vi "Channel RED.vi"() -> ()   [LabVIEW 2012]
uses:
  RxTXCamera/RxTxCamera.lvclass
  CCDCamera/CCDCamera.lvclass
  RxTx/RxTx.lvclass/RxTx.ctl
  CCDCamera/CCDCamera.lvclass/CCDCamera.ctl
  RxTXCamera/RxTxCamera.lvclass/RxTxCamera.ctl
  RxTx/Read Message.vi
  RxTXCamera/Read Construct String Header.lvclass.vi
  RxTXCamera/Write Construct String Header.lvclass.vi
  RxTXCamera/Read Construct String Setup Cam.lvclass.vi
  RxTXCamera/Write Construct String Setup Cam.lvclass.vi
  Construct String Header/Read Header Contents.vi
  Construct String Setup Cam/Read Camera Setup.vi
  Construct String Header/Construct String Header.lvclass
  Construct String Setup Cam/Construct String Setup Cam.lvclass
  RxTx/RxTx.lvclass
  Cooler/Cooler.lvclass
panel:
  in  "RxTxCamera.lvclass":refnum<class "RxTxCamera.lvclass">
  in  "error out":errorcluster
  in  "Instrument out":refnum<class "CCDCamera.lvclass">
  in  "RxTxCamera.lvclass 2":refnum<class "RxTxCamera.lvclass">
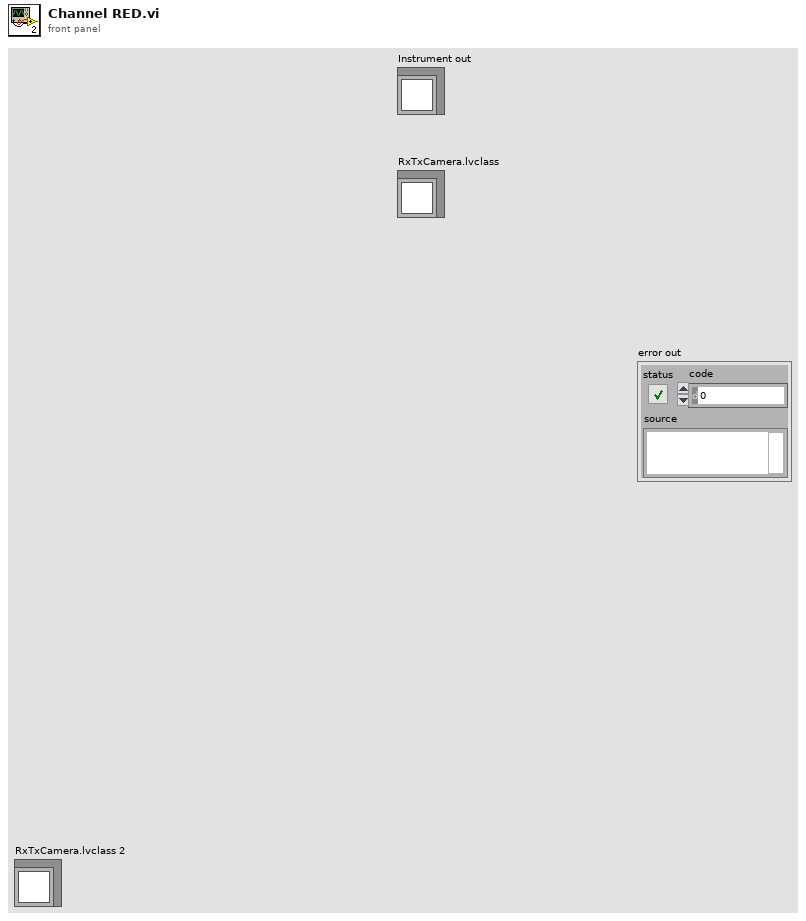
[diagram p1: front panel]
types:
  T1 = cluster{"Currently Temperature":dbl, "Last Image":string, "% Acquired":dbl, "Initilizarion":bool, "Exposing":bool, "Temperature Status":string, "X length":dbl, "Y length":dbl, "Min Temperature":dbl, "Max Temperature":dbl}
  T2 = cluster{"Cooler ON/OFF":u16, "Set temperature":dbl, "Temperature ºC":dbl, "Shutter Mode ":u16, "Shutter TTL":u16, "Time to open (ms)":dbl, "Time to close (ms)":dbl, "Baseline Clamp 2":bool, "EM Advanced 2":bool, "EM Gain  level ":i32, "EM Gain":bool, "Pre-amplifier gain":i32, "Vertical clock\n  voltage amplitude":i32, "Vertical Shift Speed":i32, "Readout Rate ":i32, "Trigger ":u16, "Conventional/EM":i32, "Read Mode ":u16, "Acquisition Mode ":u16, "Exposure Time (s) ":sgl, "XY Graph":cluster{dbl, dbl}[], "Sub Image":enum32{"256 x 256", "512 x 512", "1024 x 1024", "Custom", "128 x 128", "64 x 64"}, "Initial Line":i32, "Initial Column":i32, "Final Line":i32, "Final Column":i32, "Horizontal binning":i32, "Vertical binning ":i32, "# Exposure":u32, "Image Name":string, "Night Directory":string, "FITS Format":u16, "Image Format":string, "Tiff Position ":u16, "Tiff Type":u16}
  T3 = cluster{"Currently Temperature":dbl, "Last Image":string, "% Acquired":dbl, "Initilization":bool, "Exposing":bool, "Temperature Status":string, "X length":dbl, "Y length":dbl, "Min Temperature":dbl, "Max Temperature":dbl}
  T4 = cluster{"FILENAME":string[], "OBSERVER":string[], "PROGRID":string[], "OBJECT":string[], "NIGHTDIR":string[], "CHANNEL":string[], "INSTRUME":string[], "NEXPSEQ":string[], "SEQINDEX":string[], "OBSTYPE":string[], "READMOD":string[], "SHUTTER":string[], "OPENSHT":string[], "CLOSESHT":string[], "GAIN":string[], "GAINERR ":string[], "RDNOISE":string[], "RNOISERR":string[], "SKYFIBER":string[], "CALFIBER":string[], "UTDATE":string[], "LOCTIME":string[], "MJD":string[], "OBSLON":string[], "OBSLAT":string[], "OBSALT":string[], "EXPTIME":string[], "TELRA":string[], "TELDEC":string[], "RA":string[], "DEC":string[], "RA_DEG":string[], "DEC_DEG":string[], "EPOCH":string[], "HA":string[], "HAD":string[], "AIRMASS":string[], "AMSTART":string[], "AMEND":string[], "XOFFSET":string[], "YOFFSET":string[], "PA":string[], "CAMFOC":string[], "TELFOC":string[], "TCSUT":string[], "MOONDIST":string[], "MOONALT":string[], "MONNPHAS":string[], "ADC":string[], "ADCSPPED":string[], "CALMIRR":string[], "GUIDING":string[], "GUIDTEXP":string[], "GUIDFREQ":string[], "GUIDOBJX":string[], "GUIDOBJY":string[], "AVGYCORR":string[], "AVGXCORR":string[], "GFOCUS":string[], "THARLAMP":string[], "HALLAMP":string[], "AGITATOR":string[], "THARMIRR":string[], "DSTATUS":string[], "DTEMP":string[], "DHUM":string[], "DLAMP":string[], "DFLAT":string[], "TEMPEXT":string[], "PRESSURE":string[], "HUMIDITY":string[], "WINDDIR":string[], "WSPEED":string[], "TCSST":string[], "DPOS":string[]}
  T5 = cluster{"Acquisition Mode":u16, "Read Mode":u16, "Trigger":u16, "Conventional/EM":u16, "Shutter Mode":u16, "Shutter TTL":u16, "Time to open Shutter":u16, "Time to close Shutter":u16, "Exposure time":dbl, "Readout Rate":u16, "VShift Speed":u16, "Pre amp":u16, "Initial line":u16, "Initial column":u16, "Final column":u32, "Final line":u32, "hbin":u16, "vbin":u16, "Temperature":dbl, "Cooler ON/OFF":u16, "FITS Format":u16, "tiff position":u16, "Tiff Type":u16, "Image Format":string, "Image Path":string}
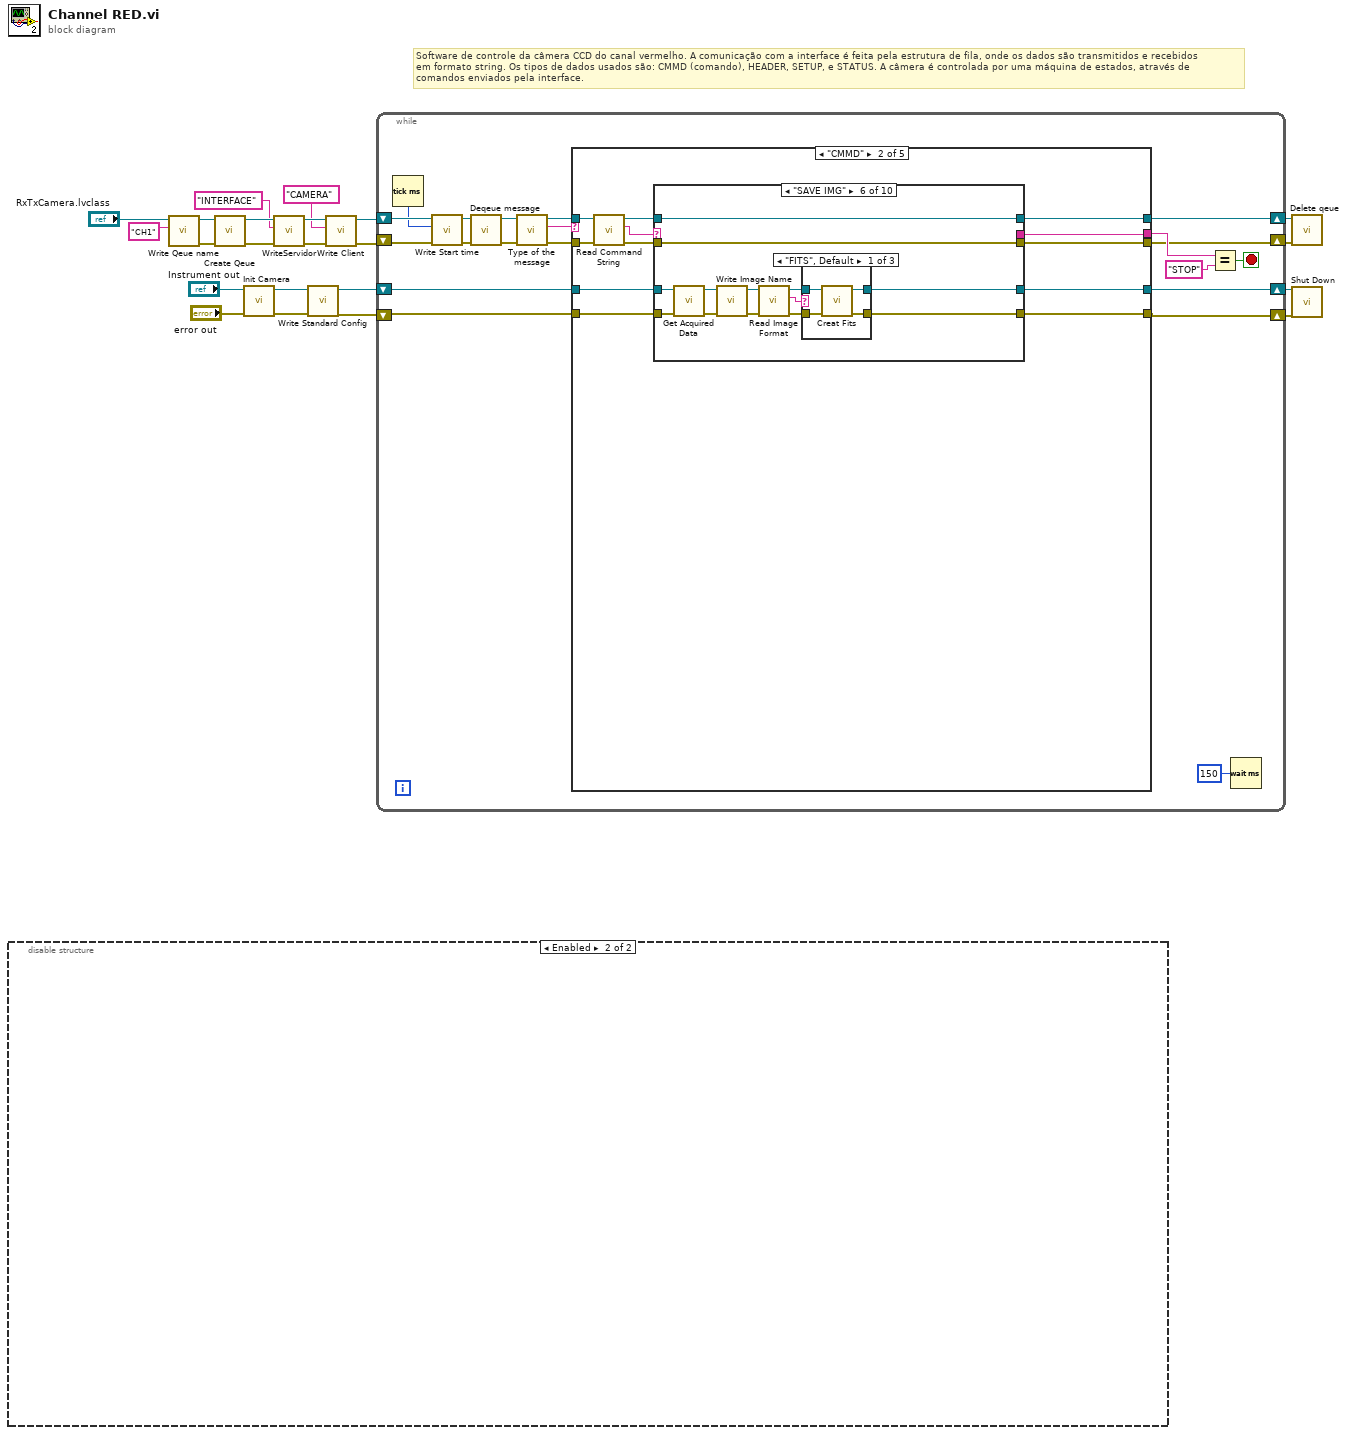
[diagram p0: block diagram]
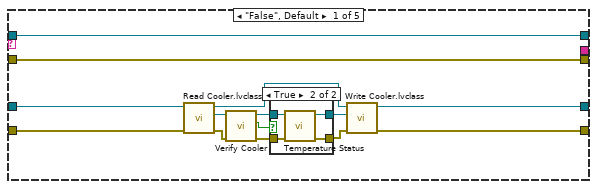
[diagram p2: hidden frame]
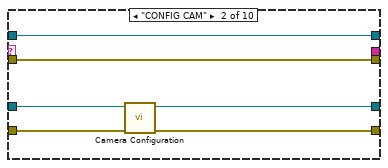
[diagram p5: hidden frame]
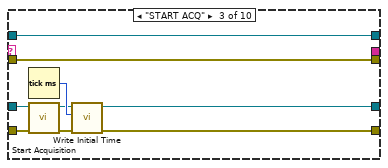
[diagram p6: hidden frame]
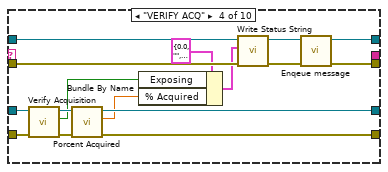
[diagram p7: hidden frame]
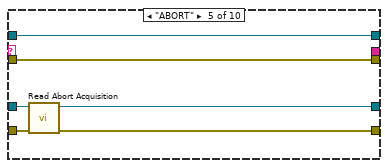
[diagram p8: hidden frame]
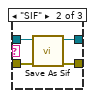
[diagram p9: hidden frame]
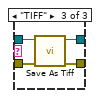
[diagram p10: hidden frame]
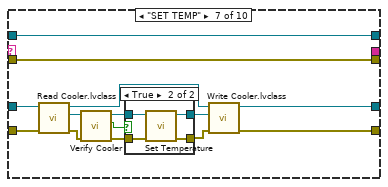
[diagram p11: hidden frame]
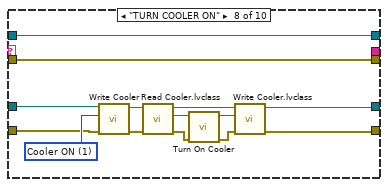
[diagram p13: hidden frame]
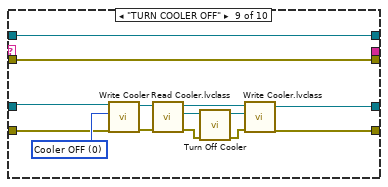
[diagram p14: hidden frame]
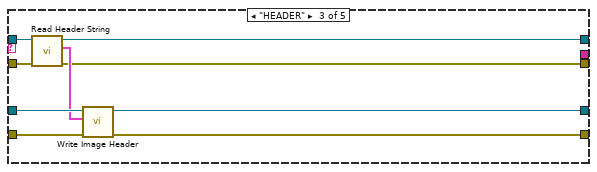
[diagram p16: hidden frame]
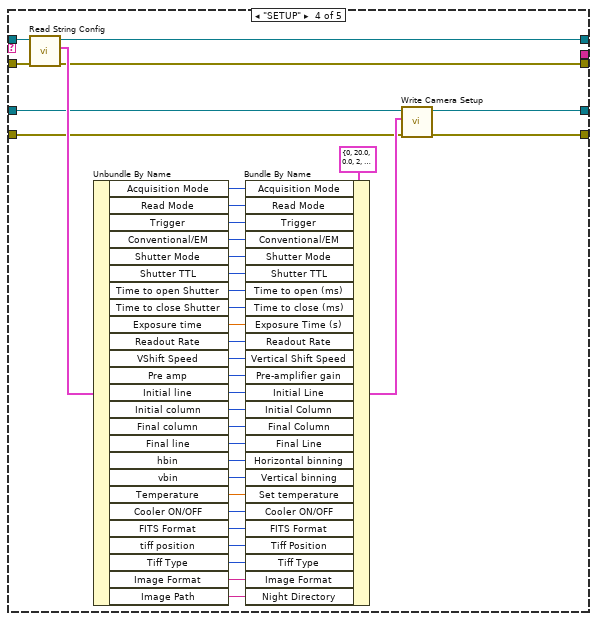
[diagram p17: hidden frame]
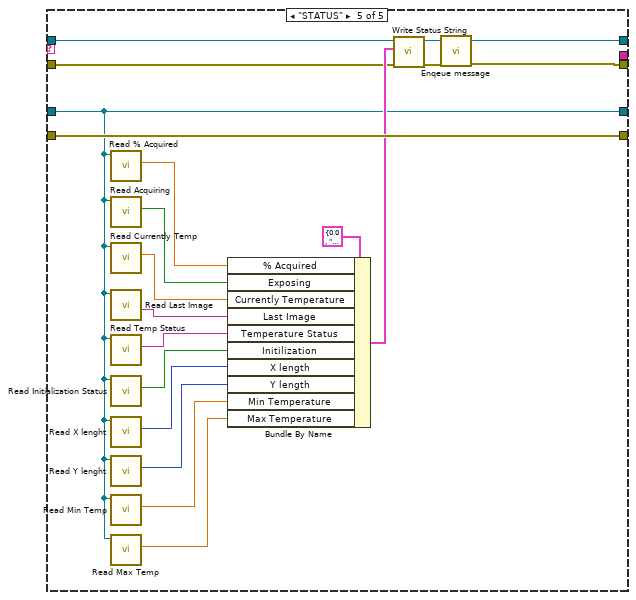
[diagram p18: hidden frame]
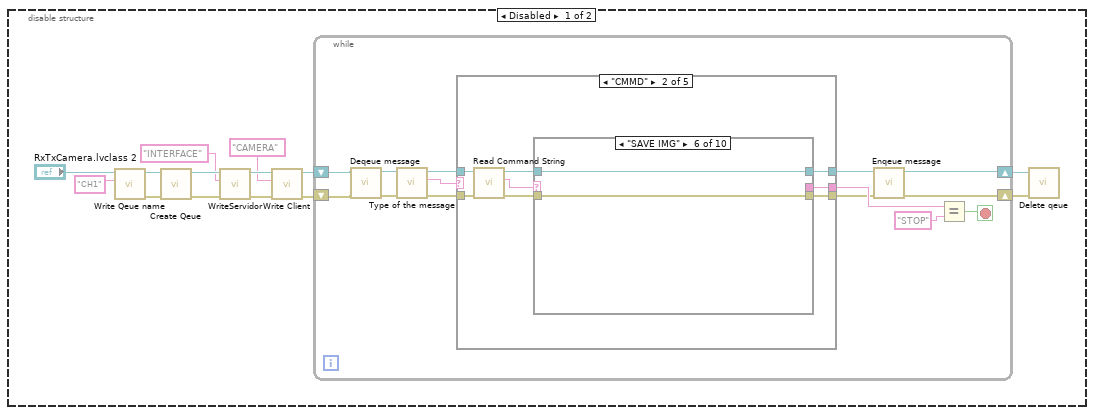
[diagram p19: hidden frame]
diagram:
  # "Software de controle da câmera CCD do canal vermelho. A comunicação com a interface é feita pela estrutura de fila, onde os dados são transmitidos e recebidos\nem formato string. Os tipos de dados usados são: CMMD (comando), HEADER, SETUP, e STATUS. A câmera é controlada por uma máquina de estados, através de\ncomandos enviados pela interface."
  n1 = disable-structure shown="Enabled" {
    frame Disabled {
      n2 = call "Write Qeue name.vi"("Qeue name"="CH1", "RxTx in"="RxTxCamera.lvclass 2") -> ("error out"=w34:errorcluster, "RxTx out"=w35:refnum<class "RxTxCamera.lvclass">)  [unwired: 8 in]
      n3 = call "Create Qeue.vi"("error in (no error)"=w34, "RxTx in"=w35) -> ("error out"=w29:errorcluster, "RxTx out"=w30:refnum<class "RxTxCamera.lvclass">)  [unwired: 8 in]
      n4 = call "WriteServidor.vi"("error in (no error)"=w29, "Servidor"="INTERFACE" ("Qeue name"), "RxTx in"=w30) -> ("error out"=w32:errorcluster, "RxTx out"=w31:refnum<class "RxTxCamera.lvclass">)  [unwired: 7 in]
      n5 = call "Write Client.vi"("error in (no error)"=w32, "Client"="CAMERA" ("Qeue name"), "RxTx in"=w31) -> ("error out"=w25:errorcluster, "RxTx out"=w26:refnum<class "RxTxCamera.lvclass">)  [unwired: 7 in]
      n6 = while {
        shift-right: [w38] -> w24
        shift-left: w25 -> [w45]
        shift-right: [w39] -> w23
        shift-left: w26 -> [w46]
        stop <- w41 stop-if-true
        n7 = call "Deqeue message.vi"("error in (no error)"=w45, "RxTx in"=w46) -> ("error out"=w50:errorcluster, "RxTx out"=w37:refnum<class "RxTxCamera.lvclass">)  [unwired: 8 in]
        n8 = call "Type of the message.vi"("error in (no error)"=w50, "RxTxCamera in"=w37) -> ("error out"=w47:errorcluster, "Type"=w40:string, "RxTxCamera out"=w48:refnum<class "RxTxCamera.lvclass">)  [unwired: 7 in]
        n9 = case shown="\"CMMD\"" w40 {
          tunnel: w48 -> [w52 w57 w89 w91 w93]
          tunnel: w47 -> [w51 w56 w88 w90 w92]
          tunnel: [w52 w55 w89 w91 w93] -> w44
          tunnel: [_ w54 _ _ _] -> w43
          tunnel: [w51 w53 w88 w90 w92] -> w42
          frame "False", Default {
          }
          frame "CMMD" {
            n10 = call "Read Command String.vi"("error in (no error)"=w56, "RxTxCamera in"=w57) -> ("error out"=w58:errorcluster, "String Command"=w60:string, "RxTxCamera out"=w59:refnum<class "RxTxCamera.lvclass">)  [unwired: 7 in]
            n11 = case shown="\"SAVE IMG\"" w60 {
              selector: w60 -> [_ _ _ _ _ _ _ _ _ w85]
              tunnel: w59 -> [w61 w63 w65 w73 w75 w77 w79 w82 w83 w87]
              tunnel: w58 -> [w62 w64 w66 w74 w76 w78 w80 w81 w84 w86]
              tunnel: [w62 w64 w66 w72 w76 w78 w80 w81 w84 w86] -> w53
              tunnel: [w61 w63 w65 w71 w75 w77 w79 w82 w83 w87] -> w55
              tunnel: [_ _ _ _ _ _ _ _ _ w85] -> w54
              frame "FALSE", Default {
              }
              frame "CONFIG CAM" {
              }
              frame "START ACQ" {
              }
              frame "VERIFY ACQ" {
                n12 = Bundle By Name(cluster=T1 {"Currently Temperature"=0.0, "Last Image"="", "% Acquired"=0.0, "Initilizarion"=FALSE, "Exposing"=FALSE, "Temperature Status"="", "X length"=0.0, "Y length"=0.0, "Min Temperature"=0.0, "Max Temperature"=0.0} ("Camera Status"), "Exposing"=FALSE, "% Acquired"=0.0) -> (w69:T1)
                n13 = call "Write Status String.vi"("error in (no error)"=w74, "Camera Status"=w69, "RxTxCamera in"=w73) -> ("error out"=w72:errorcluster, "RxTxCamera out"=w71:refnum<class "RxTxCamera.lvclass">)  [unwired: 7 in]
              }
              frame "ABORT" {
              }
              frame "SAVE IMG" {
              }
              frame "SET TEMP" {
              }
              frame "TURN COOLER ON" {
              }
              frame "TURN COOLER OFF" {
              }
              frame "STOP" {
              }
            }
          }
          frame "HEADER" {
          }
          frame "STATUS" {
          }
          frame "SETUP" {
          }
        }
        n14 = call "Enqeue message.vi"("error in (no error)"=w42, "RxTx in"=w44) -> ("error out"=w38:errorcluster, "RxTx out"=w39:refnum<class "RxTxCamera.lvclass">)  [unwired: 8 in]
        n15 = Equal?(x=w43, y="STOP") -> (x = y?=w41:bool)
      }
      n16 = call "Delete qeue.vi"("error in (no error)"=w24, "RxTx in"=w23) -> ()  [unwired: 8 in, 2 out]
    }
    frame Enabled {
    }
  }
  n17 = call "Write Qeue name.vi"("Qeue name"="CH1", "RxTx in"="RxTxCamera.lvclass") -> ("error out"=w20:errorcluster, "RxTx out"=w21:refnum<class "RxTxCamera.lvclass">)  [unwired: 8 in]
  n18 = call "Create Qeue.vi"("error in (no error)"=w20, "RxTx in"=w21) -> ("error out"=w9:errorcluster, "RxTx out"=w10:refnum<class "RxTxCamera.lvclass">)  [unwired: 8 in]
  n19 = call "Init Camera.vi"("error in (no error)"="error out", "CCDCamera in"="Instrument out") -> ("error out"=w4:errorcluster, "CCDCamera out"=w3:refnum<class "CCDCamera.lvclass">)  [unwired: 8 in]
  n20 = call "WriteServidor.vi"("error in (no error)"=w9, "Servidor"="INTERFACE" ("Qeue name"), "RxTx in"=w10) -> ("error out"=w12:errorcluster, "RxTx out"=w11:refnum<class "RxTxCamera.lvclass">)  [unwired: 7 in]
  n21 = call "Write Standard Config.vi"("error in (no error)"=w4, "CCDCamera in"=w3) -> ("error out"=w1:errorcluster, "CCDCamera out"=w2:refnum<class "CCDCamera.lvclass">)  [unwired: 8 in]
  n22 = call "Write Client.vi"("error in (no error)"=w12, "Client"="CAMERA" ("Qeue name"), "RxTx in"=w11) -> ("error out"=w5:errorcluster, "RxTx out"=w6:refnum<class "RxTxCamera.lvclass">)  [unwired: 7 in]
  n23 = while {
    shift-right: [w107] -> w14
    shift-left: w1 -> [w105]
    shift-right: [w108] -> w13
    shift-left: w2 -> [w106]
    shift-right: [w100] -> w18
    shift-left: w5 -> [w95]
    shift-right: [w99] -> w17
    shift-left: w6 -> [w96]
    stop <- w104 stop-if-true
    n24 = Tick Count (ms)() -> (millisecond timer value=w94:u32)
    n25 = call "Write Start time.vi"("error in (no error)"=w95, "Start time"=w94, "RxTx in"=w96) -> ("error out"=w98:errorcluster, "RxTx out"=w97:refnum<class "RxTxCamera.lvclass">)  [unwired: 7 in]
    n26 = call "Deqeue message.vi"("error in (no error)"=w98, "RxTx in"=w97) -> ("error out"=w113:errorcluster, "RxTx out"=w112:refnum<class "RxTxCamera.lvclass">)  [unwired: 8 in]
    n27 = call "Type of the message.vi"("error in (no error)"=w113, "RxTxCamera in"=w112) -> ("error out"=w110:errorcluster, "Type"=w111:string, "RxTxCamera out"=w109:refnum<class "RxTxCamera.lvclass">)  [unwired: 7 in]
    n28 = case shown="\"CMMD\"" w111 {
      tunnel: [w114 w145 w271 w309 w329] -> w107
      tunnel: [w116 w144 w270 w308 w319] -> w108
      tunnel: w110 -> [w127 w141 w273 w307 w320]
      tunnel: w109 -> [w126 w140 w272 w306 w321]
      tunnel: w106 -> [w117 w142 w268 w278 w319]
      tunnel: w105 -> [w115 w143 w269 w277 w329]
      tunnel: [w126 w135 w265 w276 w310] -> w99
      tunnel: [w127 w136 w266 w275 w311] -> w100
      tunnel: [_ w134 _ _ _] -> w102
      frame "False", Default {
        n29 = call "Read Cooler.lvclass.vi"("error in (no error)"=w115, "CCDCamera in"=w117) -> ("error out"=w123:errorcluster, "Cooler.lvclass"=w124:refnum<class "Cooler.lvclass">, "CCDCamera out"=w125:refnum<class "CCDCamera.lvclass">)  [unwired: 7 in]
        n30 = call "Verify Cooler.vi"("error in (no error)"=w123, "Cooler.lvclass"=w124) -> ("error out"=w119:errorcluster, "coolerStatus"=w118:bool, "Cooler.lvclass"=w120:refnum<class "Cooler.lvclass">)  [unwired: 7 in]
        n31 = case shown="True" w118 {
          tunnel: w119 -> [w128 w131]
          tunnel: w120 -> [w129 w130]
          tunnel: [w129 w133] -> w122
          tunnel: [w128 w132] -> w121
          frame False {
          }
          frame True {
            n32 = call "Temperature Status.vi"("error in (no error)"=w131, "Cooler in"=w130) -> ("error out"=w132:errorcluster, "Cooler out"=w133:refnum<class "Cooler.lvclass">)  [unwired: 8 in]
          }
        }
        n33 = call "Write Cooler.lvclass.vi"("error in (no error)"=w121, "Cooler.lvclass"=w122, "CCDCamera in"=w125) -> ("error out"=w114:errorcluster, "CCDCamera out"=w116:refnum<class "CCDCamera.lvclass">)  [unwired: 7 in]
      }
      frame "CMMD" {
        n34 = call "Read Command String.vi"("error in (no error)"=w141, "RxTxCamera in"=w140) -> ("error out"=w137:errorcluster, "String Command"=w139:string, "RxTxCamera out"=w138:refnum<class "RxTxCamera.lvclass">)  [unwired: 7 in]
        n35 = case shown="\"SAVE IMG\"" w139 {
          selector: w139 -> [_ _ _ _ _ _ _ _ _ w260]
          tunnel: [w149 w154 w160 w177 w185 w188 w215 w235 w251 w261] -> w145
          tunnel: [w148 w155 w161 w178 w186 w187 w214 w234 w250 w262] -> w144
          tunnel: w143 -> [w149 w153 w159 w175 w184 w192 w212 w233 w248 w261]
          tunnel: w142 -> [w148 w152 w158 w176 w183 w191 w213 w232 w249 w262]
          tunnel: w138 -> [w146 w150 w156 w173 w181 w189 w224 w245 w246 w264]
          tunnel: w137 -> [w147 w151 w157 w174 w182 w190 w225 w244 w247 w263]
          tunnel: [w147 w151 w157 w165 w182 w190 w225 w244 w247 w263] -> w136
          tunnel: [w146 w150 w156 w166 w181 w189 w224 w245 w246 w264] -> w135
          tunnel: [_ _ _ _ _ _ _ _ _ w260] -> w134
          frame "FALSE", Default {
          }
          frame "CONFIG CAM" {
            n36 = call "Camera Configuration.vi"("error in (no error)"=w153, "CCDCamera in"=w152) -> ("error out"=w154:errorcluster, "CCDCamera out"=w155:refnum<class "CCDCamera.lvclass">)  [unwired: 8 in]
          }
          frame "START ACQ" {
            n37 = Tick Count (ms)() -> (millisecond timer value=w164:u32)
            n38 = call "Start Acquisition.vi"("error in (no error)"=w159, "CCDCamera in"=w158) -> ("error out"=w162:errorcluster, "CCDCamera out"=w163:refnum<class "CCDCamera.lvclass">)  [unwired: 8 in]
            n39 = call "Write Initial Time.vi"("error in (no error)"=w162, "Initial Time"=w164, "CCDCamera in"=w163) -> ("error out"=w160:errorcluster, "CCDCamera out"=w161:refnum<class "CCDCamera.lvclass">)  [unwired: 7 in]
          }
          frame "VERIFY ACQ" {
            n40 = call "Verify Acquisition.vi"("error in (no error)"=w175, "CCDCamera in"=w176) -> ("error out"=w180:errorcluster, "Acquiring"=w169:bool, "CCDCamera out"=w179:refnum<class "CCDCamera.lvclass">)  [unwired: 7 in]
            n41 = call "Porcent Acquired.vi"("error in (no error)"=w180, "CCDCamera in"=w179) -> ("error out"=w177:errorcluster, "% Acquired"=w170:dbl, "CCDCamera out"=w178:refnum<class "CCDCamera.lvclass">)  [unwired: 7 in]
            n42 = Bundle By Name(cluster=T1 {"Currently Temperature"=0.0, "Last Image"="", "% Acquired"=0.0, "Initilizarion"=FALSE, "Exposing"=FALSE, "Temperature Status"="", "X length"=0.0, "Y length"=0.0, "Min Temperature"=0.0, "Max Temperature"=0.0} ("Camera Status"), "Exposing"=w169, "% Acquired"=w170) -> (w171:T1)
            n43 = call "Write Status String.vi"("error in (no error)"=w174, "Camera Status"=w171, "RxTxCamera in"=w173) -> ("error out"=w168:errorcluster, "RxTxCamera out"=w167:refnum<class "RxTxCamera.lvclass">)  [unwired: 7 in]
            n44 = call "Enqeue message.vi"("error in (no error)"=w168, "RxTx in"=w167) -> ("error out"=w165:errorcluster, "RxTx out"=w166:refnum<class "RxTxCamera.lvclass">)  [unwired: 8 in]
          }
          frame "ABORT" {
            n45 = call "Read Abort Acquisition.vi"("error in (no error)"=w184, "CCDCamera in"=w183) -> ("error out"=w185:errorcluster, "CCDCamera out"=w186:refnum<class "CCDCamera.lvclass">)  [unwired: 7 in, 1 out]
          }
          frame "SAVE IMG" {
            n46 = call "Get Acquired Data.vi"("error in (no error)"=w192, "CCDCamera in"=w191) -> ("error out"=w199:errorcluster, "CCDCamera out"=w198:refnum<class "CCDCamera.lvclass">)  [unwired: 8 in]
            n47 = call "Write Image Name.vi"("error in (no error)"=w199, "CCDCamera in"=w198) -> ("error out"=w197:errorcluster, "CCDCamera out"=w196:refnum<class "CCDCamera.lvclass">)  [unwired: 8 in]
            n48 = call "Read Image Format.vi"("error in (no error)"=w197, "CCDCamera in"=w196) -> ("error out"=w193:errorcluster, "Image Format"=w195:string, "CCDCamera out"=w194:refnum<class "CCDCamera.lvclass">)  [unwired: 7 in]
            n49 = case shown="\"FITS\", Default" w195 {
              tunnel: w194 -> [w202 w206 w211]
              tunnel: w193 -> [w203 w207 w210]
              tunnel: [w201 w205 w208] -> w187
              tunnel: [w200 w204 w209] -> w188
              frame "FITS", Default {
                n50 = call "Creat Fits.vi"("error in (no error)"=w203, "CCDCamera in"=w202) -> ("error out"=w200:errorcluster, "CCDCamera out"=w201:refnum<class "CCDCamera.lvclass">)  [unwired: 8 in]
              }
              frame "SIF" {
                n51 = call "Save As Sif.vi"("error in (no error)"=w207, "CCDCamera in"=w206) -> ("error out"=w204:errorcluster, "CCDCamera out"=w205:refnum<class "CCDCamera.lvclass">)  [unwired: 8 in]
              }
              frame "TIFF" {
                n52 = call "Save As Tiff.vi"("error in (no error)"=w210, "CCDCamera in"=w211) -> ("error out"=w209:errorcluster, "CCDCamera out"=w208:refnum<class "CCDCamera.lvclass">)  [unwired: 8 in]
              }
            }
          }
          frame "SET TEMP" {
            n53 = call "Read Cooler.lvclass.vi"("error in (no error)"=w212, "CCDCamera in"=w213) -> ("error out"=w221:errorcluster, "Cooler.lvclass"=w222:refnum<class "Cooler.lvclass">, "CCDCamera out"=w223:refnum<class "CCDCamera.lvclass">)  [unwired: 7 in]
            n54 = call "Verify Cooler.vi"("error in (no error)"=w221, "Cooler.lvclass"=w222) -> ("error out"=w217:errorcluster, "coolerStatus"=w216:bool, "Cooler.lvclass"=w218:refnum<class "Cooler.lvclass">)  [unwired: 7 in]
            n55 = case shown="True" w216 {
              tunnel: w217 -> [w226 w231]
              tunnel: w218 -> [w227 w230]
              tunnel: [w227 w229] -> w220
              tunnel: [w226 w228] -> w219
              frame False {
              }
              frame True {
                n56 = call "Set Temperature.vi"("error in (no error)"=w231, "Cooler in"=w230) -> ("error out"=w228:errorcluster, "Cooler out"=w229:refnum<class "Cooler.lvclass">)  [unwired: 8 in]
              }
            }
            n57 = call "Write Cooler.lvclass.vi"("error in (no error)"=w219, "Cooler.lvclass"=w220, "CCDCamera in"=w223) -> ("error out"=w215:errorcluster, "CCDCamera out"=w214:refnum<class "CCDCamera.lvclass">)  [unwired: 7 in]
          }
          frame "TURN COOLER ON" {
            w243 = u16 1 items=["Cooler OFF", "Cooler ON"] ("Cooler ON/OFF")
            n58 = call "Write Cooler.vi"("error in (no error)"=w233, "Cooler ON/OFF"=w243, "CCDCamera in"=w232) -> ("error out"=w236:errorcluster, "CCDCamera out"=w242:refnum<class "CCDCamera.lvclass">)  [unwired: 7 in]
            n59 = call "Read Cooler.lvclass.vi"("error in (no error)"=w236, "CCDCamera in"=w242) -> ("error out"=w237:errorcluster, "Cooler.lvclass"=w240:refnum<class "Cooler.lvclass">, "CCDCamera out"=w241:refnum<class "CCDCamera.lvclass">)  [unwired: 7 in]
            n60 = call "Turn On Cooler.vi"("error in (no error)"=w237, "Cooler in"=w240) -> ("error out"=w238:errorcluster, "Cooler out"=w239:refnum<class "Cooler.lvclass">)  [unwired: 8 in]
            n61 = call "Write Cooler.lvclass.vi"("error in (no error)"=w238, "Cooler.lvclass"=w239, "CCDCamera in"=w241) -> ("error out"=w235:errorcluster, "CCDCamera out"=w234:refnum<class "CCDCamera.lvclass">)  [unwired: 7 in]
          }
          frame "TURN COOLER OFF" {
            w255 = u16 0 items=["Cooler OFF", "Cooler ON"] ("Cooler ON/OFF")
            n62 = call "Write Cooler.vi"("error in (no error)"=w248, "Cooler ON/OFF"=w255, "CCDCamera in"=w249) -> ("error out"=w252:errorcluster, "CCDCamera out"=w254:refnum<class "CCDCamera.lvclass">)  [unwired: 7 in]
            n63 = call "Read Cooler.lvclass.vi"("error in (no error)"=w252, "CCDCamera in"=w254) -> ("error out"=w259:errorcluster, "Cooler.lvclass"=w258:refnum<class "Cooler.lvclass">, "CCDCamera out"=w253:refnum<class "CCDCamera.lvclass">)  [unwired: 7 in]
            n64 = call "Turn Off Cooler.vi"("error in (no error)"=w259, "Cooler in"=w258) -> ("error out"=w256:errorcluster, "Cooler out"=w257:refnum<class "Cooler.lvclass">)  [unwired: 8 in]
            n65 = call "Write Cooler.lvclass.vi"("error in (no error)"=w256, "Cooler.lvclass"=w257, "CCDCamera in"=w253) -> ("error out"=w251:errorcluster, "CCDCamera out"=w250:refnum<class "CCDCamera.lvclass">)  [unwired: 7 in]
          }
          frame "STOP" {
          }
        }
      }
      frame "HEADER" {
        n66 = call "Read Header String.vi"("error in (no error)"=w273, "RxTxCamera in"=w272) -> ("error out"=w266:errorcluster, "Header Contents"=w267:T4, "RxTxCamera out"=w265:refnum<class "RxTxCamera.lvclass">)  [unwired: 7 in]
        n67 = call "Write Image Header.vi"("error in (no error)"=w269, "Header Contents"=w267, "CCDCamera in"=w268) -> ("error out"=w271:errorcluster, "CCDCamera out"=w270:refnum<class "CCDCamera.lvclass">)  [unwired: 7 in]
      }
      frame "SETUP" {
        n68 = call "Read String Config.vi"("error in (no error)"=w307, "RxTxCamera in"=w306) -> ("error out"=w275:errorcluster, "Camera Setup"=w305:T5, "RxTxCamera out"=w276:refnum<class "RxTxCamera.lvclass">)  [unwired: 7 in]
        n69 = Unbundle By Name(w305) -> ("Acquisition Mode"=w280:u16, "Read Mode"=w281:u16, "Trigger"=w282:u16, "Conventional/EM"=w283:u16, "Shutter Mode"=w284:u16, "Shutter TTL"=w285:u16, "Time to open Shutter"=w286:u16, "Time to close Shutter"=w287:u16, "Exposure time"=w288:dbl, "Readout Rate"=w289:u16, "VShift Speed"=w290:u16, "Pre amp"=w291:u16, "Initial line"=w292:u16, "Initial column"=w293:u16, "Final column"=w294:u32, "Final line"=w295:u32, "hbin"=w296:u16, "vbin"=w297:u16, "Temperature"=w298:dbl, "Cooler ON/OFF"=w299:u16, "FITS Format"=w300:u16, "tiff position"=w301:u16, "Tiff Type"=w302:u16, "Image Format"=w303:string, "Image Path"=w274:string)
        n70 = Bundle By Name(cluster=T2 {"Cooler ON/OFF"=0, "Set temperature"=20.0, "Temperature ºC"=0.0, "Shutter Mode "=2, "Shutter TTL"=0, "Time to open (ms)"=50.0, "Time to close (ms)"=50.0, "Baseline Clamp 2"=FALSE, "EM Advanced 2"=FALSE, "EM Gain  level "=1, "EM Gain"=FALSE, "Pre-amplifier gain"=1, "Vertical clock\n  voltage amplitude"=0, "Vertical Shift Speed"=0, "Readout Rate "=0, "Trigger "=0, "Conventional/EM"=1, "Read Mode "=4, "Acquisition Mode "=1, "Exposure Time (s) "=0.0, "XY Graph"=[], "Sub Image"=enum."1024 x 1024", "Initial Line"=1, "Initial Column"=1, "Final Line"=1, "Final Column"=1, "Horizontal binning"=1, "Vertical binning "=1, "# Exposure"=1, "Image Name"="", "Night Directory"="", "FITS Format"=0, "Image Format"="", "Tiff Position "=1, "Tiff Type"=0} ("RED Channel Settings"), "Acquisition Mode"=w280, "Read Mode"=w281, "Trigger"=w282, "Conventional/EM"=w283, "Shutter Mode"=w284, "Shutter TTL"=w285, "Time to open (ms)"=w286, "Time to close (ms)"=w287, "Exposure Time (s)"=w288, "Readout Rate"=w289, "Vertical Shift Speed"=w290, "Pre-amplifier gain"=w291, "Initial Line"=w292, "Initial Column"=w293, "Final Column"=w294, "Final Line"=w295, "Horizontal binning"=w296, "Vertical binning"=w297, "Set temperature"=w298, "Cooler ON/OFF"=w299, "FITS Format"=w300, "Tiff Position"=w301, "Tiff Type"=w302, "Image Format"=w303, "Night Directory"=w274) -> (w279:T2)
        n71 = call "Write Camera Setup.vi"("error in (no error)"=w277, "RED Channel Settings"=w279, "CCDCamera in"=w278) -> ("error out"=w309:errorcluster, "CCDCamera out"=w308:refnum<class "CCDCamera.lvclass">)  [unwired: 7 in]
      }
      frame "STATUS" {
        n72 = call "Read % Acquired.vi"("CCDCamera in"=w319) -> ("% Acquired"=w328:dbl)  [unwired: 8 in, 2 out]
        n73 = call "Read Acquiring.vi"("CCDCamera in"=w319) -> ("Acquiring"=w327:bool)  [unwired: 8 in, 2 out]
        n74 = call "Read Currently Temp.vi"("CCDCamera in"=w319) -> ("Currently Temp"=w326:dbl)  [unwired: 8 in, 2 out]
        n75 = call "Read Last Image.vi"("CCDCamera in"=w319) -> ("Last Image"=w325:string)  [unwired: 7 in, 3 out]
        n76 = call "Read Temp Status.vi"("CCDCamera in"=w319) -> ("Temp Status"=w324:string)  [unwired: 8 in, 2 out]
        n77 = call "Read Initialization Status.vi"("CCDCamera in"=w319) -> ("Initialization Status"=w323:bool)  [unwired: 8 in, 2 out]
        n78 = call "Read X lenght.vi"("CCDCamera in"=w319) -> ("X lenght"=w318:u16)  [unwired: 8 in, 2 out]
        n79 = call "Read Y lenght.vi"("CCDCamera in"=w319) -> ("Y lenght"=w317:u16)  [unwired: 8 in, 2 out]
        n80 = call "Read Min Temp.vi"("CCDCamera in"=w319) -> ("Min Temp"=w316:dbl)  [unwired: 8 in, 2 out]
        n81 = call "Read Max Temp.vi"("CCDCamera in"=w319) -> ("Max Temp"=w315:dbl)  [unwired: 8 in, 2 out]
        n82 = Bundle By Name(cluster=T3 {"Currently Temperature"=0.0, "Last Image"="", "% Acquired"=0.0, "Initilization"=FALSE, "Exposing"=FALSE, "Temperature Status"="", "X length"=0.0, "Y length"=0.0, "Min Temperature"=0.0, "Max Temperature"=0.0} ("Camera Status"), "% Acquired"=w328, "Exposing"=w327, "Currently Temperature"=w326, "Last Image"=w325, "Temperature Status"=w324, "Initilization"=w323, "X length"=w318, "Y length"=w317, "Min Temperature"=w316, "Max Temperature"=w315) -> (w322:T3)
        n83 = call "Write Status String.vi"("error in (no error)"=w320, "Camera Status"=w322, "RxTxCamera in"=w321) -> ("error out"=w313:errorcluster, "RxTxCamera out"=w312:refnum<class "RxTxCamera.lvclass">)  [unwired: 7 in]
        n84 = call "Enqeue message.vi"("error in (no error)"=w313, "RxTx in"=w312) -> ("error out"=w311:errorcluster, "RxTx out"=w310:refnum<class "RxTxCamera.lvclass">)  [unwired: 8 in]
      }
    }
    n85 = Equal?(x=w102, y="STOP") -> (x = y?=w104:bool)
    n86 = Wait (ms)(milliseconds to wait=u32 150) -> ()  [unwired: 1 out]
  }
  n87 = call "Delete qeue.vi"("error in (no error)"=w18, "RxTx in"=w17) -> ()  [unwired: 8 in, 2 out]
  n88 = call "Shut Down.vi"("error in (no error)"=w14, "CCDCamera in"=w13) -> ()  [unwired: 8 in, 2 out]
